vi "example3.vi"() -> ()   [LabVIEW 2018, in "LV-Julia_ZMQ-Roundtrip_lib.lvlib"]
uses:
  LV-Julia_ZMQ-Roundtrip_lib.lvlib
  Julia functions enum.ctl
  example args cluster.ctl
  example server response cluster.ctl
  Commands v2.ctl
  <vilib>/Analysis/baseanly.llb/Mean (DBL).vi
  <vilib>/Analysis/NI_AALBase.lvlib
panel:
  out "parsed response":T1 {"bin_lng" format="%.0e"}
  out "sample size":i32
  in  "bindata size":u32
  out "min value":dbl
  out "max value":dbl
  out "median":dbl format="%.6f"
  out "mean":dbl format="%.5f"
  out "final error":errorcluster
  out "current error":errorcluster
  out "status":string
  in  "stop":bool
  out "roundtrip time":dbl
  in  "Arguments":T2={"arg1"=1, "arg2"=3.14}
  in  "fun2call":T3
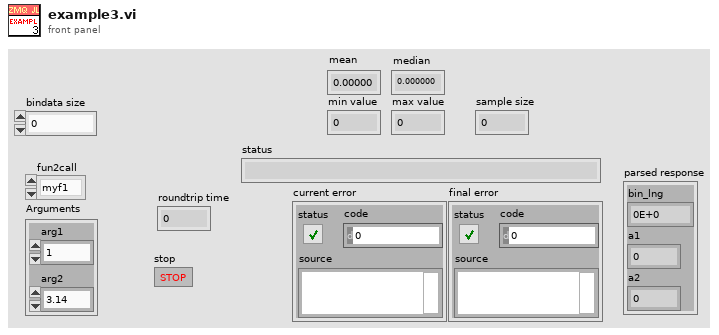
[diagram p1: front panel]
types:
  T1 = typedef "example server response cluster.ctl" = cluster{"bin_lng":i32, "a1":i32, "a2":dbl}
  T2 = typedef "example args cluster.ctl" = cluster{"arg1":i32, "arg2":dbl}
  T3 = typedef "Julia functions enum.ctl" = enum16{"myf1", "myf2", "myf3"}
  T4 = typedef "LV-Julia_ZMQ-Roundtrip_lib.lvlib/Commands v2.ctl" = enum16{"Start Jl-server & Init LV-client", "Send request & Get response ", "Stop Jl-server & Cleanup LV-client", "Cleanup LV-client", "Start Jl-server", "Stop Jl-server", "Init LV-Client", "Cleanup LV-Client", "(not allowed)", "Set LV Client state", "Set Jl Server state"}
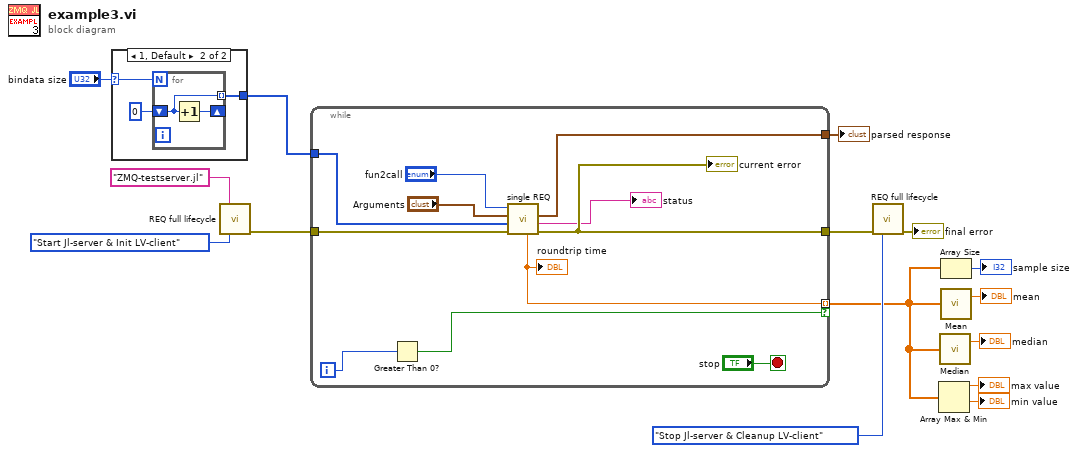
[diagram p0: block diagram]
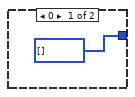
[diagram p2: hidden frame]
diagram:
  n1 = case shown="1, Default" "bindata size" {
    selector: "bindata size" -> [_ w19]
    tunnel: [u8[] [] w17] -> w4
    frame 0 {
    }
    frame 1, Default {
      n2 = for {
        N: w19 -> [_]
        shift-right: [w21] -> _
        shift-left: u8 0 -> [w20]
        tunnel: [w20] -> w17 mode=indexing
        n3 = Increment(x=w20) -> (x+1=w21:u8)
      }
    }
  }
  n4 = call "REQ full lifecycle.vi"("Julia ZMQ server file name"="ZMQ-testserver.jl", "command"=Commands_v2."Start Jl-server & Init LV-client") -> ("error out"=w15:errorcluster)  [unwired: 10 in, 3 out]
  n5 = while {
    tunnel: w15 -> [w32]
    tunnel: [w31] -> w14
    tunnel: [w26] -> w3 mode=indexing if=w24
    tunnel: w4 -> [w23]
    tunnel: [w22] -> w1
    i -> [w25]
    stop <- "stop" stop-if-true
    n6 = Greater Than 0?(x=w25) -> (x > 0?=w24:bool)
    n7 = call "single REQ.vi"("error in (no error)"=w32, "binary data in"=w23, "Arguments"="Arguments", "fun2call"="fun2call") -> ("error out"=w31:errorcluster, "detailed err description or other information"=→"status":string, "parsed response"=w22:T1, "roundtrip time"=w26:dbl)  [unwired: 3 in, 1 out]
    "roundtrip time" <- w26
    "current error" <- w31
  }
  "parsed response" <- w1
  n8 = call "REQ full lifecycle.vi"("error in"=w14, "command"=Commands_v2."Stop Jl-server & Cleanup LV-client") -> ("error out"=→"final error":errorcluster)  [unwired: 10 in, 3 out]
  n9 = Array Max & Min(array=w3) -> (max value=→"max value":dbl, min value=→"min value":dbl)  [unwired: 2 out]
  n10 = call <vilib>:"Median.vi"("X"=w3) -> ("median"=→"median":dbl)  [unwired: 1 out]
  n11 = Array Size(array=w3) -> (size(s)=→"sample size":i32)
  n12 = call-poly <vilib>:"Mean.vi"("X"=w3) -> ("mean"=→"mean":dbl)  [unwired: 1 out]
